vi "make_code_verifier.vi"(8 "error in (no error)":errorcluster, 11 "size":i32=43) -> (0 "error out":errorcluster, 3 "code_verifier":string)   [LabVIEW 2015, in "lv-dropbox.lvlib"]
uses:
  lv-dropbox.lvlib
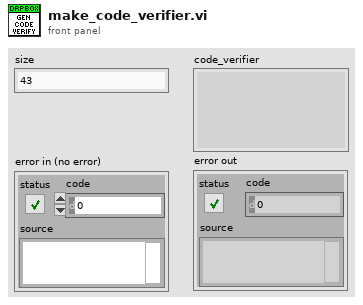
[diagram p1: front panel]
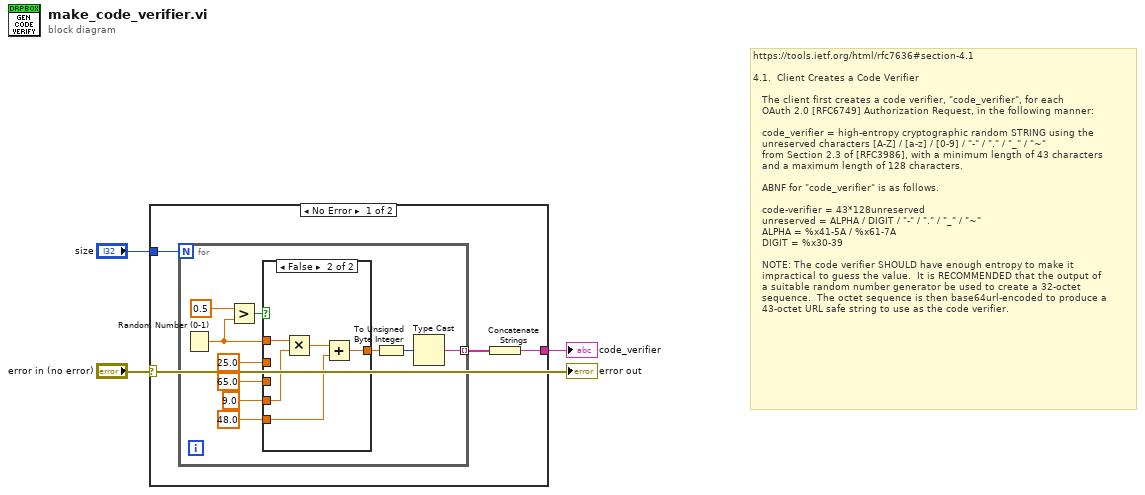
[diagram p0: block diagram]
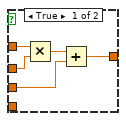
[diagram p2: hidden frame]
diagram:
  # "https://tools.ietf.org/html/rfc7636#section-4.1\n\n4.1.  Client Creates a Code Verifier\n\n   The client first creates a code verifier, \"code_verifier\", for each\n   OAuth 2.0 [RFC6749] Authorization Request, in the following manner:\n\n   code_verifier = high-entropy cryptographic random STRING using the\n   unreserved characters [A-Z] / [a-z] / [0-9] / \"-\" / \".\" / \"_\" / \"~\"\n   from Section 2.3 of [RFC3986], with a minimum length of 43 characters\n   and a maximum length of 128 characters.\n\n   ABNF for \"code_verifier\" is as follows.\n\n   code-verifier = 43*128unreserved\n   unreserved = ALPHA / DIGIT / \"-\" / \".\" / \"_\" / \"~\"\n   ALPHA = %x41-5A / %x61-7A\n   DIGIT = %x30-39\n\n   NOTE: The code verifier SHOULD have enough entropy to make it\n   impractical to guess the value.  It is RECOMMENDED that the output of\n   a suitable random number generator be used to create a 32-octet\n   sequence.  The octet sequence is then base64url-encoded to produce a\n   43-octet URL safe string to use as the code verifier."
  n1 = case shown="No Error" "error in (no error)" {
    tunnel: "size" -> [w6 _]
    tunnel: [w4 _] -> w2
    frame No Error {
      n2 = for {
        N: w6 -> [_]
        tunnel: [w14] -> w5 mode=indexing
        n3 = Random Number (0-1)() -> (number: 0 to 1=w11:dbl)
        n4 = Greater?(x=0.5, y=w11) -> (0:w13:bool)
        n5 = case shown="False" w13 {
          tunnel: w11 -> [w21 w26]
          tunnel: [w19 w24] -> w16
          tunnel: 25.0 ("y") -> [w18 _]
          tunnel: 65.0 ("y") -> [w17 _]
          tunnel: 9.0 ("y") -> [_ w23]
          tunnel: 48.0 ("y") -> [_ w22]
          frame True {
            n6 = Multiply(x=w21, y=w18) -> (x*y=w20:dbl)
            n7 = Add(x=w20, y=w17) -> (x+y=w19:dbl)
          }
          frame False {
            n8 = Multiply(x=w26, y=w23) -> (x*y=w25:dbl)
            n9 = Add(x=w25, y=w22) -> (x+y=w24:dbl)
          }
        }
        n10 = To Unsigned Byte Integer(number=w16) -> (unsigned 8bit integer=w15:u8)
        n11 = Type Cast(x=w15) -> (*(type *) &x=w14:string)  [unwired: 1 in]
      }
      n12 = Concatenate Strings(w5) -> (w4:string)
    }
    frame Error {
    }
  }
  "code_verifier" <- w2
  "error out" <- "error in (no error)"
